vi "Delete scan settings.vi"(8 "Path":path, 11 "Scan settings name":string) -> (0 "error out":errorcluster)   [LabVIEW 2011]
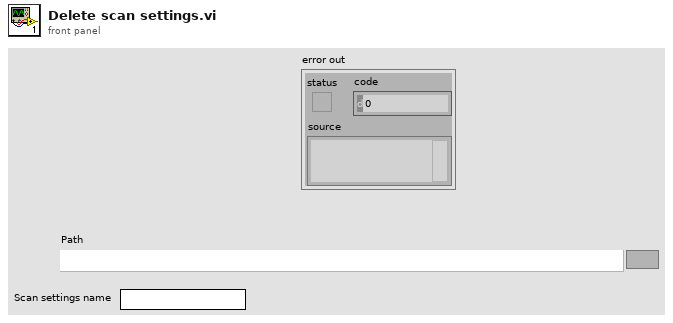
[diagram p1: front panel]
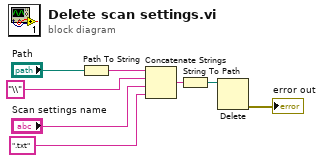
[diagram p0: block diagram]
diagram:
  n1 = Path To String(path="Path") -> (string=w8:string)
  n2 = Concatenate Strings(w8, "\\", "Scan settings name", ".txt" ("y")) -> (w7:string)
  n3 = String To Path(string=w7) -> (path=w2:path)
  n4 = Delete(path (use dialog)=w2) -> (error out=→"error out":errorcluster)  [unwired: 4 in, 2 out]
